vi "Get Data.vi"(11 "Audit Event":refnum<class "Audit Event.lvclass">) -> (3 "Audit Event":T1)   [LabVIEW 2026, in "Audit Event.lvclass"]
uses:
  Audit Event.lvclass
  Audit Event.lvclass/Audit Event.ctl
  Typedefs/enums/Audit Event Type Enum.ctl
  Typedefs/clusters/Audit Event Data.ctl
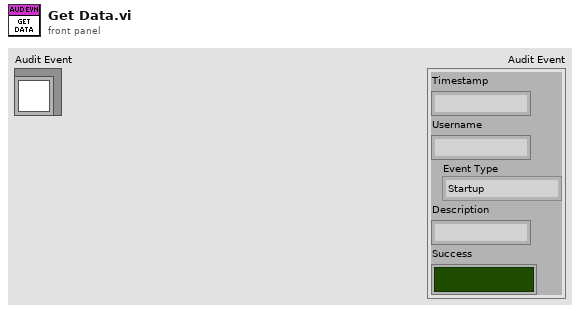
[diagram p1: front panel]
types:
  T1 = typedef "Audit Event Data.ctl" = cluster{"Timestamp":string, "Username":string, "Event Type":T2, "Description":string, "Success":bool}
  T2 = typedef "Audit Event Type Enum.ctl" = enum16{"Startup", "Shutdown", "Login", "Logout", "ReadinessCheck", "RunStarted", "RunFinished", "Error"}
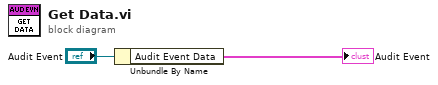
[diagram p0: block diagram]
diagram:
  n1 = Unbundle By Name("Audit Event") -> ("Audit Event Data"=→"Audit Event":T1)
